vi "specu1a 1.0.0 Read PUnit Information.vi"(3 "error in (no error)":errorcluster, 5 "Device Handle":i32) -> (0 "error out":errorcluster, 1 "Unit Information out":T1={"UnitID"="", "Sensor Name"="", "Serial Number"="", "Reserved"="", "Wave Upper"=630, "Wave Lower"=1050}, 2 "Device Handle out":i32)   [LabVIEW 2019]
uses:
  Controls/specu1a 1.0.0 Product Information.ctl
  specu1a.dll
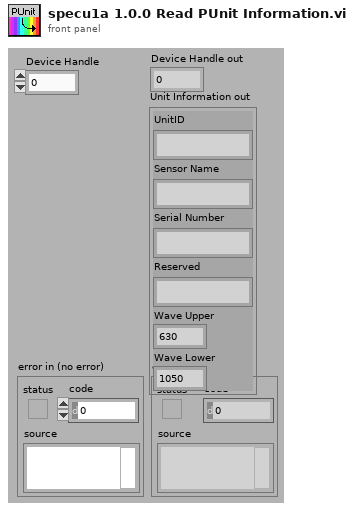
[diagram p1: front panel]
types:
  T1 = typedef "specu1a 1.0.0 Product Information.ctl" = cluster{"UnitID":string, "Sensor Name":string, "Serial Number":string, "Reserved":string, "Wave Upper":u16, "Wave Lower":u16}
  T2 = cluster{"UnitID":cluster{u8, u8, u8, u8, u8, u8, u8, u8}, "Sensor Name":cluster{u8, u8, u8, u8, u8, u8, u8, u8, u8, u8, u8, u8, u8, u8, u8, u8}, "Serial Number":cluster{u8, u8, u8, u8, u8, u8, u8, u8}, "Reserved":cluster{u8, u8, u8, u8, u8, u8, u8, u8}, "Wave Upper":u16, "Wave Lower":u16}
  T3 = typedef "specu1a 1.0.0 Error codes.ctl" = enum16{"INVALID_HANDLE_VALUE", "USBDEV_SUCCESS", "USBDEV_INVALID_HANDLE", "USBDEV_UNSUCCESS", "USBDEV_INVALID_VALUE", "USBDEV_CHECK_NORMAL", "USBDEV_CHECK_INVALID", "USBDEV_CHECK_REMOVE", "USBDEV_CHECK_OTHER", "USBDEV_RESET_ERROR", "USBDEV_BULKSIZE_ERROR", "USBDEV_BULK_READ_ERROR", "USBDEV_BULK_NOT_UPDATED", "USBDEV_TIME_OVER_ERROR", "USBDEV_TIME_UNDER_ERROR", "USBDEV_TIME_SET_ERROR", "USBDEV_SET_GAIN_ERROR", "USBDEV_GET_TEMP_ERROR", "USBDEV_SET_TRIGGER_ERROR", "USBDEV_RW_EEP_ADDR_ERROR", "USBDEV_RW_EEP_SIZE_ERROR", "USBDEV_RW_EEP_OVER_ERROR", "USBDEV_RW_EEP_ERROR", "UNITID_PRODUCTID_CONFLICT", "UNKNOWN_ERROR"}
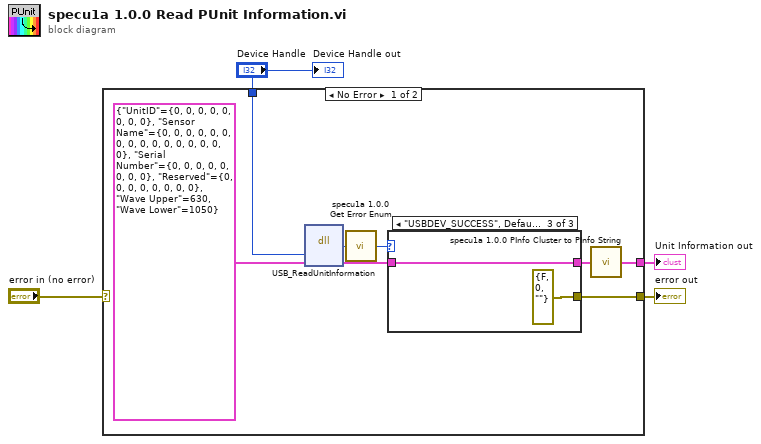
[diagram p0: block diagram]
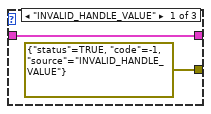
[diagram p2: hidden frame]
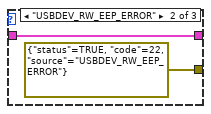
[diagram p3: hidden frame]
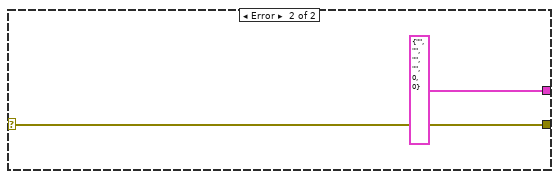
[diagram p4: hidden frame]
diagram:
  n1 = case shown="No Error" "error in (no error)" {
    selector: "error in (no error)" -> [_ w20]
    tunnel: [w8 w20] -> w3
    tunnel: [w6 T1 {"UnitID"="", "Sensor Name"="", "Serial Number"="", "Reserved"="", "Wave Upper"=0, "Wave Lower"=0} ("output cluster 2")] -> w2
    tunnel: "Device Handle" -> [w5 _]
    frame No Error {
      n2 = dll-call lib="C:/Users/martzlab/Desktop/SIO 179/Nitrate/64/EvaluationSoftware/minispec labview/Hamamatsu Spectrometer Dll/specu1a.dll" fn="USB_ReadUnitInformation" label="1.0.0 Read unit information"("Device Handle"=w5, "output cluster"=T2 {"UnitID"={0, 0, 0, 0, 0, 0, 0, 0}, "Sensor Name"={0, 0, 0, 0, 0, 0, 0, 0, 0, 0, 0, 0, 0, 0, 0, 0}, "Serial Number"={0, 0, 0, 0, 0, 0, 0, 0}, "Reserved"={0, 0, 0, 0, 0, 0, 0, 0}, "Wave Upper"=630, "Wave Lower"=1050}) -> (w11:u16, "output cluster"=w9:T2)  [unwired: 4 in, 2 out]
      n3 = call "specu1a 1.0.0 Get Error Enum.vi"("Error Code in"=w11) -> ("Specu1a 1.0.0 Error code out"=w10:T3)  [unwired: 4 in]
      n4 = case shown="\"USBDEV_SUCCESS\", Default" w10 {
        tunnel: [w13 w15 w17] -> w7
        tunnel: [errorcluster {"status"=TRUE, "code"=-1, "source"="INVALID_HANDLE_VALUE"} ("error out") errorcluster {"status"=TRUE, "code"=22, "source"="USBDEV_RW_EEP_ERROR"} ("error out") errorcluster {"status"=FALSE, "code"=0, "source"=""} ("error out")] -> w8
        tunnel: w9 -> [w13 w15 w17]
        frame "INVALID_HANDLE_VALUE" {
        }
        frame "USBDEV_RW_EEP_ERROR" {
        }
        frame "USBDEV_SUCCESS", Default {
        }
      }
      n5 = call "specu1a 1.0.0 PInfo Cluster to PInfo String.vi"("output cluster"=w7) -> ("output cluster 2"=w6:T1)
    }
    frame Error {
    }
  }
  "error out" <- w3
  "Unit Information out" <- w2
  "Device Handle out" <- "Device Handle"
